vi "Single Acquisition.vi"() -> (0 "Out (UnSigned)":fxp<+,12,12>, 2 "Out":fxp<+/-,12,12>)   [LabVIEW 2014]
doc: "Performs a single acquisition from digital pin DIO 0 to DIO 11 and returns a 12-bit FXP"
uses:
  <vilib>/rvi/eio/common/nirviEmuTemplateMethod_errors.vi
  <vilib>/eio/EIONode/EIONode.xnode
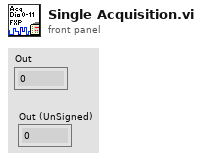
[diagram p1: front panel]
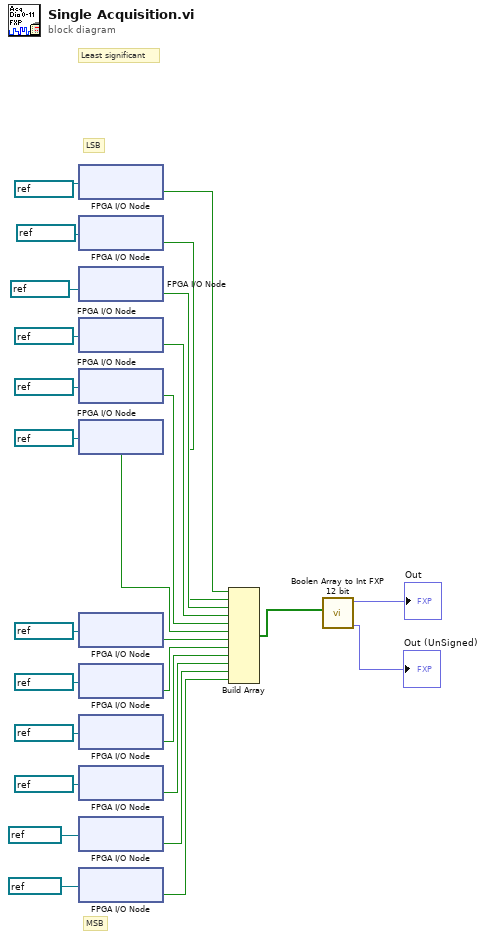
[diagram p0: block diagram]
diagram:
  # "MSB"
  # "LSB"
  # "Least significant"
  n1 = xnode "FPGA I/O Node"("FPGA I/O In"=refnum<k21> "DIO18") -> ("I/O Item"=w5:bool)  [unwired: 1 out]
  n2 = xnode "FPGA I/O Node"("FPGA I/O In"=refnum<k21> "DIO19") -> ("I/O Item"=w4:bool)  [unwired: 1 out]
  n3 = xnode "FPGA I/O Node"("FPGA I/O In"=refnum<k21> "DIO20") -> ("I/O Item"=w7:bool)  [unwired: 1 out]
  n4 = xnode "FPGA I/O Node"("FPGA I/O In"=refnum<k21> "DIO21") -> ("I/O Item"=w6:bool)  [unwired: 1 out]
  n5 = xnode "FPGA I/O Node"("FPGA I/O In"=refnum<k21> "DIO22") -> ("I/O Item"=w25:bool)  [unwired: 1 out]
  n6 = xnode "FPGA I/O Node"("FPGA I/O In"=refnum<k21> "DIO23") -> ("I/O Item"=w24:bool)  [unwired: 1 out]
  n7 = xnode "FPGA I/O Node"("FPGA I/O In"=refnum<k21> "DIO24") -> ("I/O Item"=w23:bool)  [unwired: 1 out]
  n8 = xnode "FPGA I/O Node"("FPGA I/O In"=refnum<k21> "DIO25") -> ("I/O Item"=w22:bool)  [unwired: 1 out]
  n9 = xnode "FPGA I/O Node"("FPGA I/O In"=refnum<k21> "DIO26") -> ("I/O Item"=w21:bool)  [unwired: 1 out]
  n10 = xnode "FPGA I/O Node"("FPGA I/O In"=refnum<k21> "DIO27") -> ("I/O Item"=w20:bool)  [unwired: 1 out]
  n11 = xnode "FPGA I/O Node"("FPGA I/O In"=refnum<k21> "DIO3") -> ("I/O Item"=w19:bool)  [unwired: 1 out]
  n12 = xnode "FPGA I/O Node"("FPGA I/O In"=refnum<k21> "DIO2") -> ("I/O Item"=w18:bool)  [unwired: 1 out]
  n13 = Build Array(w5, w4, w7, w6, w25, w24, w23, w22, w21, w20, w19, w18) -> (w3:bool[])
  n14 = call "Boolen Array to Int FXP 12 bit.vi"("Boolean array"=w3) -> ("UNSigned"=→"Out (UnSigned)":fxp<+,12,12>, "Signed"=→"Out":fxp<+/-,12,12>)  [unwired: 9 in]
